vi "errorHandlerTCP.vi"(7 "show popup":bool, 8 "error in":errorcluster, 9 "language":i32, 10 "error number":i8, 11 "connection ID":refnum<k5>) -> (0 "error out":errorcluster, 3 "connection ID":refnum<k5>)   [LabVIEW 2016, in "AMC_VIs.lvlib"]
uses:
  AMC_VIs.lvlib
panel:
  out "params_cluster":cluster{"language":i32, "errNbr":i32}
  in  "Params_cluster":cluster{"integer":i32, "integer":i32}
  in  "results_cluster":cluster{"errNo":i32, "string":string}
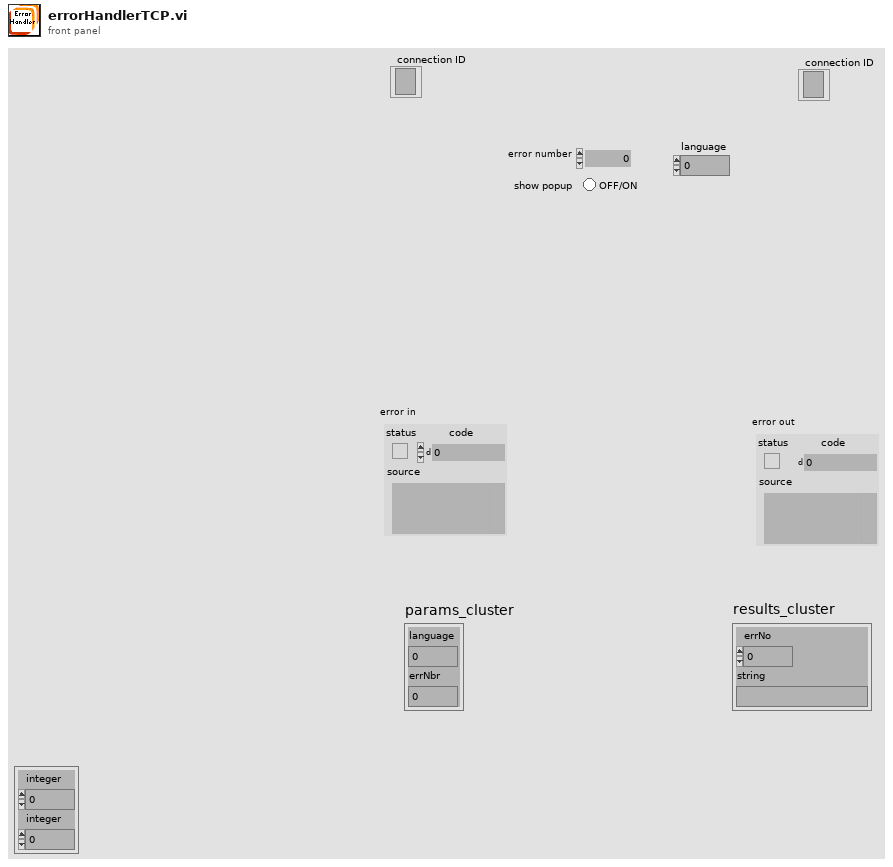
[diagram p1: front panel]
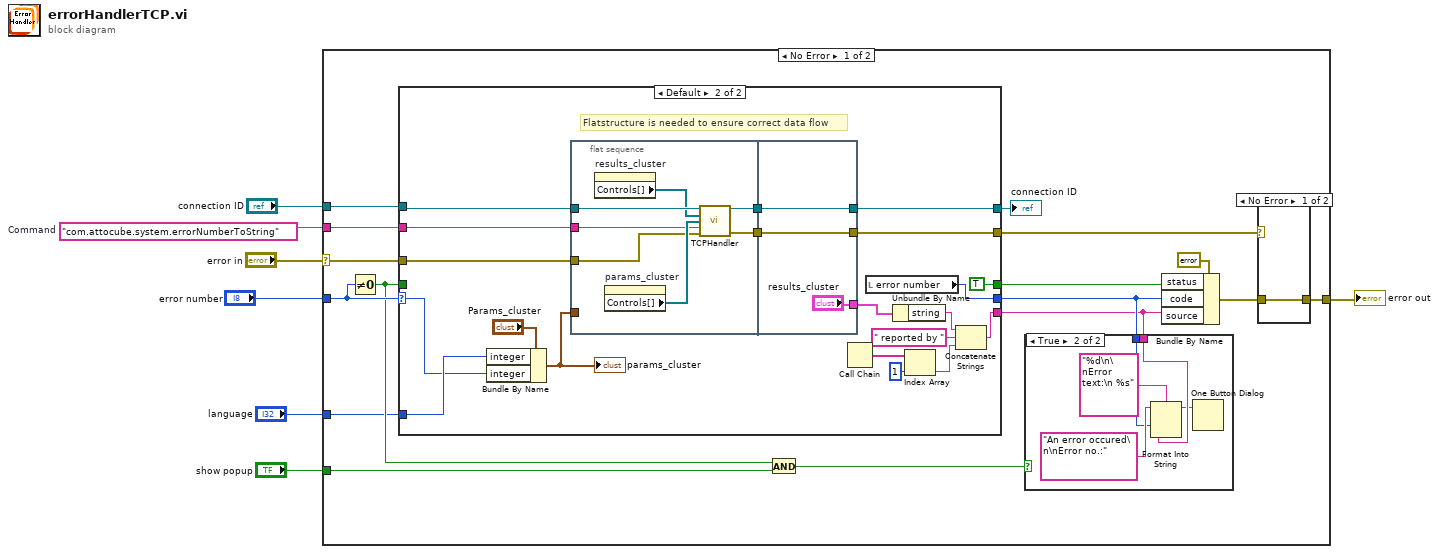
[diagram p0: block diagram]
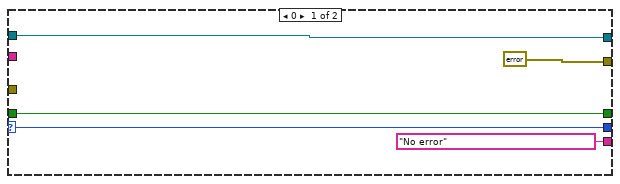
[diagram p4: hidden frame]
diagram:
  w1 = "com.attocube.system.errorNumberToString"  # Command
  n1 = case shown="No Error" "error in" {
    selector: "error in" -> [w9 w66]
    tunnel: "error number" -> [w23 _]
    tunnel: "show popup" -> [w18 _]
    tunnel: "language" -> [w16 _]
    tunnel: [w10 w66] -> w4
    tunnel: "connection ID" -> [w13 _]
    tunnel: w1 -> [w8 _]
    frame No Error {
      n2 = Not Equal To 0?(x=w23) -> (x != 0?=w19:bool)
      n3 = case shown="Default" w23 {
        selector: w23 -> [w34 w48]
        tunnel: ["No error" w36] -> w20
        tunnel: [w34 w42] -> w21
        tunnel: [w33 TRUE] -> w22
        tunnel: w19 -> [w33 _]
        tunnel: w16 -> [_ w49]
        tunnel: w13 -> [w32 w47]
        tunnel: [w32 w46] -> w15
        tunnel: [errorcluster {"status"=FALSE, "code"=0, "source"=""} ("error in") w45] -> w12
        tunnel: w9 -> [_ w44]
        tunnel: w8 -> [_ w43]
        frame 0 {
        }
        frame Default {
          # "Flatstructure is needed to ensure correct data flow"
          n4 = Bundle By Name(cluster="Params_cluster", "integer"=w49, "integer"=w48) -> (w50:cluster{"integer":i32, "integer":i32})
          "params_cluster" <- w50
          n5 = flat-sequence {
            tunnel: [w61] -> w54
            tunnel: w47 -> [w62]
            tunnel: w43 -> [w58]
            tunnel: [w57] -> w53
            tunnel: w50 -> [_]
            tunnel: w44 -> [w56]
            tunnel: ["results_cluster"] -> w52
            tunnel: [w65] -> w46
            tunnel: w54 -> [w65]
            tunnel: [w63] -> w45
            tunnel: w53 -> [w63]
            frame #0 {
              n6 = property on="results_cluster" class="Clust (strict)"() -> ("Controls[]"=w60:refnum<vi>[])  [unwired: 2 in, 2 out]
              n7 = property on="params_cluster" class="Clust (strict)"() -> ("Controls[]"=w59:refnum<vi>[])  [unwired: 2 in, 2 out]
              n8 = call "TCPHandler.vi"("connection ID"=w62, "results_cluster"=w60, "params_cluster"=w59, "method"=w58, "error"=w56) -> ("connection ID"=w61:refnum<k5>, "error"=w57:errorcluster)  [unwired: 7 in, 2 out]
            }
            frame #1 {
            }
          }
          n9 = Call Chain() -> (call chain=w41:string[])
          n10 = local read "error number"() -> (w42:i8)
          n11 = Unbundle By Name(w52) -> ("string"=w37:string)
          n12 = Index Array(array=w41, index=1) -> (element=w39:string)
          n13 = Concatenate Strings(w37, " reported by " ("string"), w39) -> (w36:string)
        }
      }
      "connection ID" <- w15
      n14 = And(x=w19, y=w18) -> (x .and. y?=w17:bool)
      n15 = case shown="True" w17 {
        tunnel: w21 -> [_ w29]
        tunnel: w20 -> [_ w27]
        frame False {
        }
        frame True {
          n16 = Format Into String(format string="%d\n\nError text:\n %s", initial string="An error occured\n\nError no.:", w29, w27) -> (resulting string=w26:string)  [unwired: 1 in, 1 out]
          n17 = One Button Dialog(message=w26) -> ()  [unwired: 1 in, 1 out]
        }
      }
      n18 = Bundle By Name(cluster=errorcluster {"status"=FALSE, "code"=0, "source"=""} ("error in"), "status"=w22, "code"=w21, "source"=w20) -> (w11:errorcluster)
      n19 = case shown="No Error" w12 {
        selector: w12 -> [_ w25]
        tunnel: w11 -> [w24 _]
        tunnel: [w24 w25] -> w10
        frame No Error {
        }
        frame Error {
        }
      }
    }
    frame Error {
    }
  }
  "error out" <- w4
